vi "Array Average.vi"(11 "data":dbl[](array[numeric])) -> (3 "Numeric":dbl)   [LabVIEW 2017]
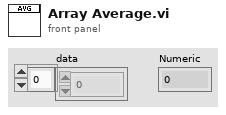
[diagram p1: front panel]
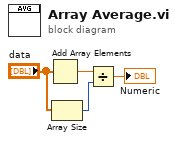
[diagram p0: block diagram]
diagram:
  n1 = Add Array Elements(numeric array="data") -> (sum=w2:dbl)
  n2 = Array Size(array="data") -> (size(s)=w1:i32)
  n3 = Divide(x=w2, y=w1) -> (x/y=→"Numeric":dbl)
